vi "sort.volume.issues.vi"(10 "issues":T3[](array[typedef]), 11 "volume data":T1) -> (3 "volume out":T1)   [LabVIEW 2024]
uses:
  CV_Shared_Library/volume.type--enum.ctl
  CV_Shared_Library/CV_Shared_Library.lvlib
  comic_manager/manager_daemon/type_defs/VolumeData--cluster.ctl
  comic_manager/manager_daemon/manager_daemon.lvclass
  comic_manager/manager_daemon/type_defs/IssueData--clustrer.ctl
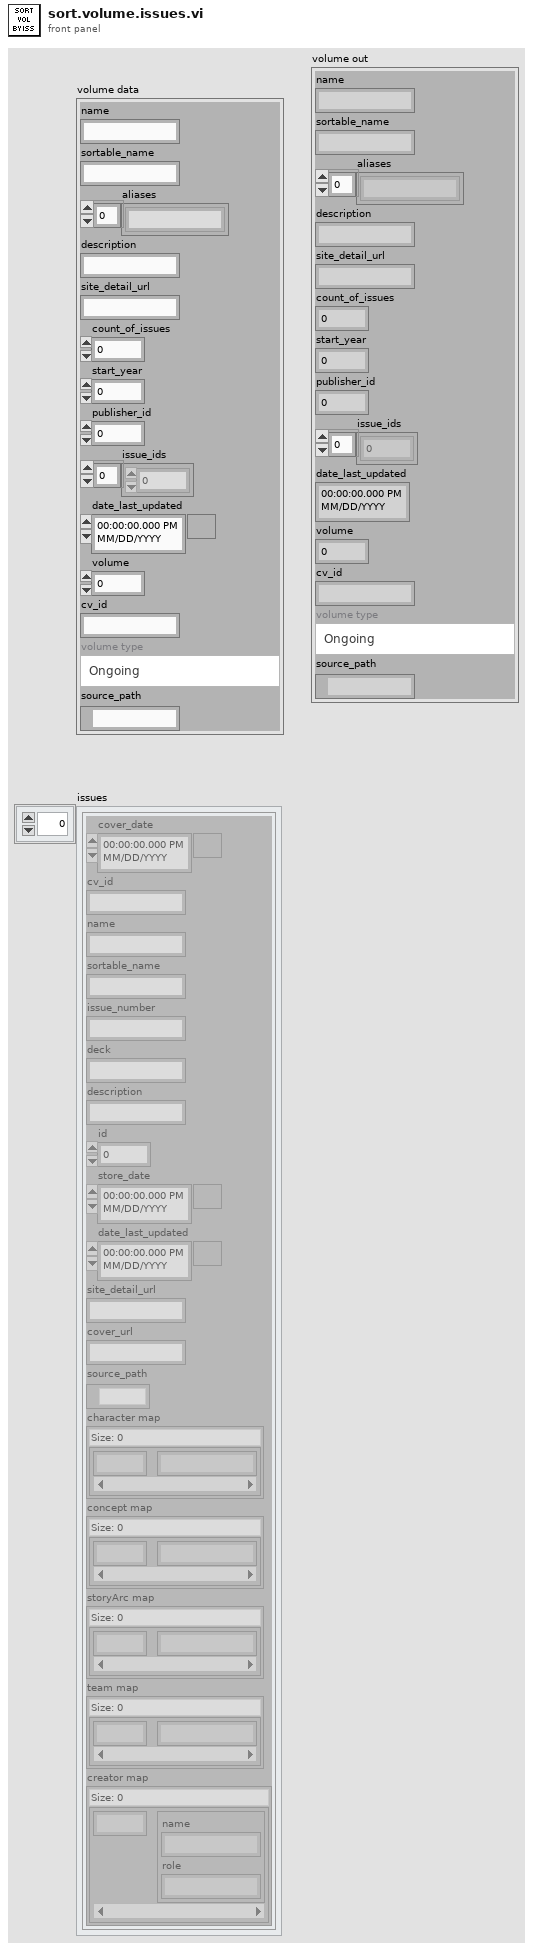
[diagram p1: front panel]
types:
  T1 = typedef "manager_daemon.lvclass/VolumeData--cluster.ctl" = cluster{"name":string, "sortable_name":string, "aliases":string[], "description":string, "site_detail_url":string, "count_of_issues":i32, "start_year":i32, "publisher_id":i32, "issue_ids":i32[], "date_last_updated":timestamp, "volume":i32, "cv_id":string, "volume type":T2, "source_path":path}
  T2 = typedef "CV_Shared_Library.lvlib/volume.type--enum.ctl" = enum16{"Ongoing", "Limited Series", "Annual", "One Shot", "Reprint/Document", "Star Comics", "Epic Comics"}
  T3 = typedef "manager_daemon.lvclass/IssueData--clustrer.ctl" = cluster{"cover_date":timestamp, "cv_id":string, "name":string, "sortable_name":string, "issue_number":string, "deck":string, "description":string, "id":i32, "store_date":timestamp, "date_last_updated":timestamp, "site_detail_url":string, "cover_url":string, "source_path":path, "character map":map{i32, string}, "concept map":map{i32, string}, "storyArc map":map{i32, string}, "team map":map{i32, string}, "creator map":map{i32, cluster{"name":string, "role":string}}}
  T4 = cluster{dbl, "issue_id":i32, "issue_number":string}
  T5 = cluster{dbl, "issue_id":i32, "issue_number":string}[]
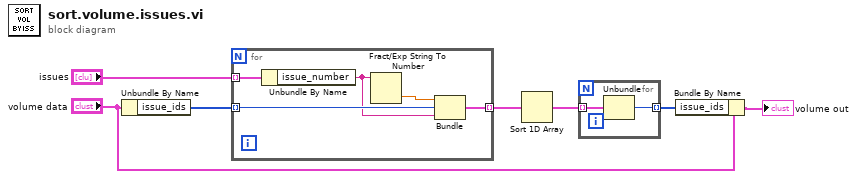
[diagram p0: block diagram]
diagram:
  n1 = Unbundle By Name("volume data") -> ("issue_ids"=w7:i32[])
  n2 = for {
    tunnel: w7 -> [w11] mode=indexing
    tunnel: "issues" -> [w8] mode=indexing
    tunnel: [w10] -> w5 mode=indexing
    n3 = Unbundle By Name(w8) -> ("issue_number"=w9:string)
    n4 = Fract/Exp String To Number(string=w9) -> (number=w12:dbl)  [unwired: 3 in, 1 out]
    n5 = Bundle(w12, "issue_id"=w11, "issue_number"=w9) -> (w10:T4)  [unwired: 1 in]
  }
  n6 = Sort 1D Array(array=w5) -> (sorted array=w3:T5)
  n7 = for {
    tunnel: w3 -> [w14] mode=indexing
    tunnel: [w13] -> w4 mode=indexing
    n8 = Unbundle(w14) -> ("issue_id"=w13:i32)  [unwired: 2 out]
  }
  n9 = Bundle By Name(cluster="volume data", "issue_ids"=w4) -> (→"volume out":T1)
